vi "Get Routing Channel State-Value Table.vi"(8 "error in":errorcluster, 11 "routing channel in":T1 format="%.0x") -> (0 "error out":errorcluster, 1 "state values":i32[](array[numeric]), 2 "state names":string[](array[string]), 3 "routing channel out":T1=18446744073709551615 format="%.0x")   [LabVIEW 2017, in "Routing and Faulting Scripting.lvlib"]
uses:
  Routing and Faulting Scripting.lvlib
  <vilib>/NI Veristand/Custom Device API/Custom Device Item Ref.ctl
  NationalInstruments.VeriStand.SystemDefinitionAPI
  NationalInstruments.VeriStand.SystemStorage
  Shared/Routing and Faulting Shared.lvlib
  <vilib>/NI Veristand/Custom Device API/Custom Device API.lvlib
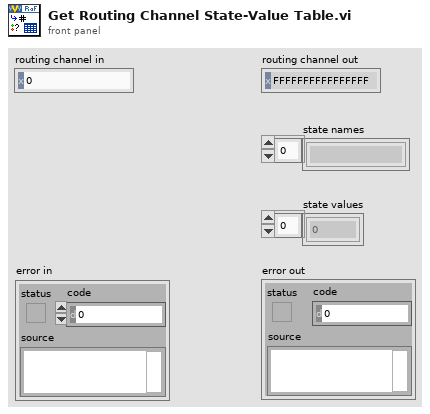
[diagram p1: front panel]
types:
  T1 = typedef "Custom Device API.lvlib/Custom Device Item Ref.ctl" = u64
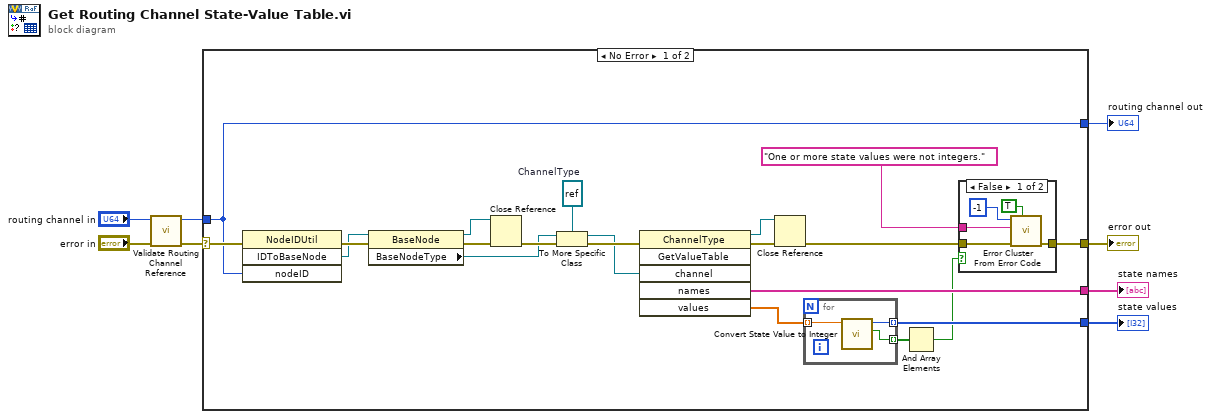
[diagram p0: block diagram]
diagram:
  n1 = call "Validate Routing Channel Reference.vi"("error in"="error in", "routing channel in"="routing channel in") -> ("error out"=w3:errorcluster, "routing channel out"=w1:T1)  [unwired: 8 in]
  n2 = case shown="No Error" w3 {
    selector: w3 -> [w26 w40]
    tunnel: [w10 w40] -> w7
    tunnel: w1 -> [w25 w39]
    tunnel: [w25 w39] -> w6
    tunnel: [w17 _] -> w5
    tunnel: [w14 _] -> w4
    frame No Error {
      w23 = refnum<k24> refnum  # ChannelType
      n3 = invoke class="NodeIDUtil" method="IDToBaseNode"(error in=w26, "nodeID"=w25) -> (error out=w29:errorcluster, "IDToBaseNode"=w27:refnum<k24>)  [unwired: 2 in, 2 out]
      n4 = property class="BaseNode"(reference=w27, error in=w29) -> (reference out=w16:refnum<k24>, error out=w28:errorcluster, "BaseNodeType"=w20:refnum<k24>)
      n5 = Close Reference(reference=w16, error in (no error)=w28) -> (error out=w21:errorcluster)
      n6 = To More Specific Class(target class=w23, reference=w20, error in=w21) -> (specific class reference=w22:refnum<k24>, error out=w24:errorcluster)
      n7 = invoke class="ChannelType" method="GetValueTable"(error in=w24, "channel"=w22) -> (reference out=w18:refnum<k24>, error out=w19:errorcluster, "names"=w17:string[], "values"=w15:dbl[])  [unwired: 4 in, 2 out]
      n8 = Close Reference(reference=w18, error in (no error)=w19) -> (error out=w11:errorcluster)
      n9 = for {
        tunnel: w15 -> [w38] mode=indexing
        tunnel: [w37] -> w14 mode=indexing
        tunnel: [w36] -> w13 mode=indexing
        n10 = call "Convert State Value to Integer.vi"("Floating Point State Value"=w38) -> ("Valid State Value"=w36:bool, "Integer State Value"=w37:i32)  [unwired: 9 in]
      }
      n11 = And Array Elements(Boolean array=w13) -> (logical AND=w12:bool)
      n12 = case shown="False" w12 {
        tunnel: w11 -> [w34 w35]
        tunnel: [w33 w35] -> w10
        tunnel: "One or more state values were not integers." ("error message (\"\")") -> [w30 _]
        frame False {
          n13 = call <vilib>:"Error Cluster From Error Code.vi"("show call chain? (False)"=TRUE, "error in (no error)"=w34, "error message (\"\")"=w30, "error code (0)"=-1) -> ("error out"=w33:errorcluster)  [unwired: 5 in]
        }
        frame True {
        }
      }
    }
    frame Error {
    }
  }
  "routing channel out" <- w6
  "error out" <- w7
  "state names" <- w5
  "state values" <- w4
